vi "Read number_of_tactics.vi"(8 "error in (no error)":errorcluster, 11 "TableFinalizerRole in":refnum<class "TableFinalizerRole.lvclass">) -> (0 "error out":errorcluster, 2 "number_of_tactics":dbl=4.0, 3 "TableFinalizerRole out":refnum<class "TableFinalizerRole.lvclass">)   [LabVIEW 2023, in "TableFinalizerRole.lvclass"]
uses:
  TableFinalizerRole.lvclass
  TableFinalizerRole.lvclass/TableFinalizerRole.ctl
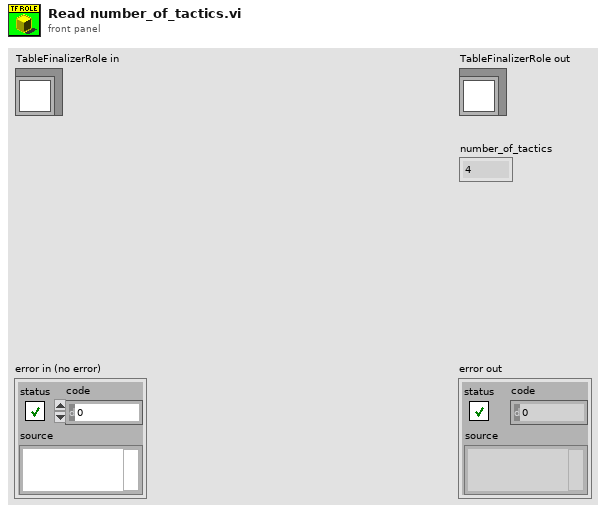
[diagram p1: front panel]
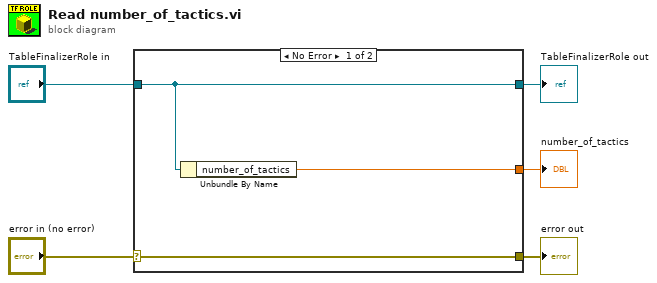
[diagram p0: block diagram]
diagram:
  n1 = case shown="No Error" "error in (no error)" {
    selector: "error in (no error)" -> [w8 w9]
    tunnel: [w8 w9] -> w4
    tunnel: [w7 w10] -> w2
    tunnel: "TableFinalizerRole in" -> [w7 w10]
    tunnel: [w6 _] -> w1
    frame No Error {
      n2 = Unbundle By Name(w7) -> ("number_of_tactics"=w6:dbl)
    }
    frame Error {
    }
  }
  "error out" <- w4
  "TableFinalizerRole out" <- w2
  "number_of_tactics" <- w1
